vi "filename-manage.vi"(6 "filename pattern":T2, 7 "filename-action":T1=enum."parse", 9 "folder IN":path=path "C:/data/Ultrasound/birdcage/Hg1201/Test", 10 "string IN":string="^(\\s+)(\\d+)_(.*)_(\\d\\d\\d\\d\\d\\d)\\.dat$", 11 "file name IN":string="f027_lsco2_122317.dat") -> (0 "number OUT":dbl=10.0 format="%#_10f", 1 "string OUT":string="^(\\s+)(\\d+)_(.*)_(\\d\\d\\d\\d\\d\\d)\\.dat$", 3 "filename OUT":string)   [LabVIEW 2021]
uses:
  filename-pattern.ctl
  filename-action.ctl
  <vilib>/Utility/libraryn.llb/Check if File or Folder Exists.vi
  <vilib>/regexp/Match Regular Expression.xnode
panel:
  out "offset past match":i32=-1
  out "whole match":string
  out "unique index out":i32
  out "pattern":string="^(\\s+)(\\d+)_(.*)_(\\d\\d\\d\\d\\d\\d)\\.dat$"
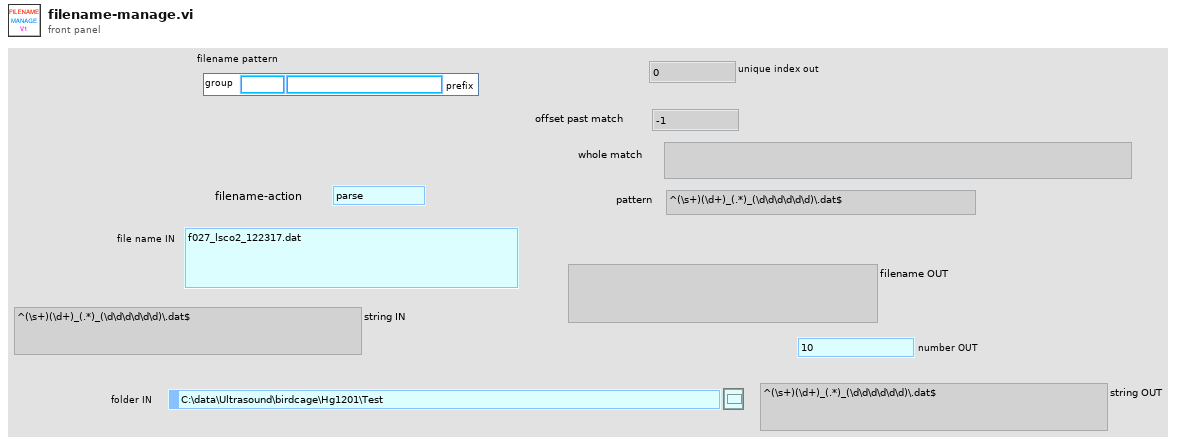
[diagram p1: front panel]
types:
  T1 = typedef "filename-action.ctl" = enum16{"rewrite", "parse", "force pattern", "uniquenum", "get T", "get B", "get ind", "get deg", "get name", "get folder", "get extension", "get basename", "get side", "get setof", "getID", "getIDStock", "remove prefix", "get36thing", "getplain", "getvproj", "getIDStanf", "remove p_c?_"}
  T2 = typedef "filename-pattern.ctl" = cluster{"prefix":string, "group":string}
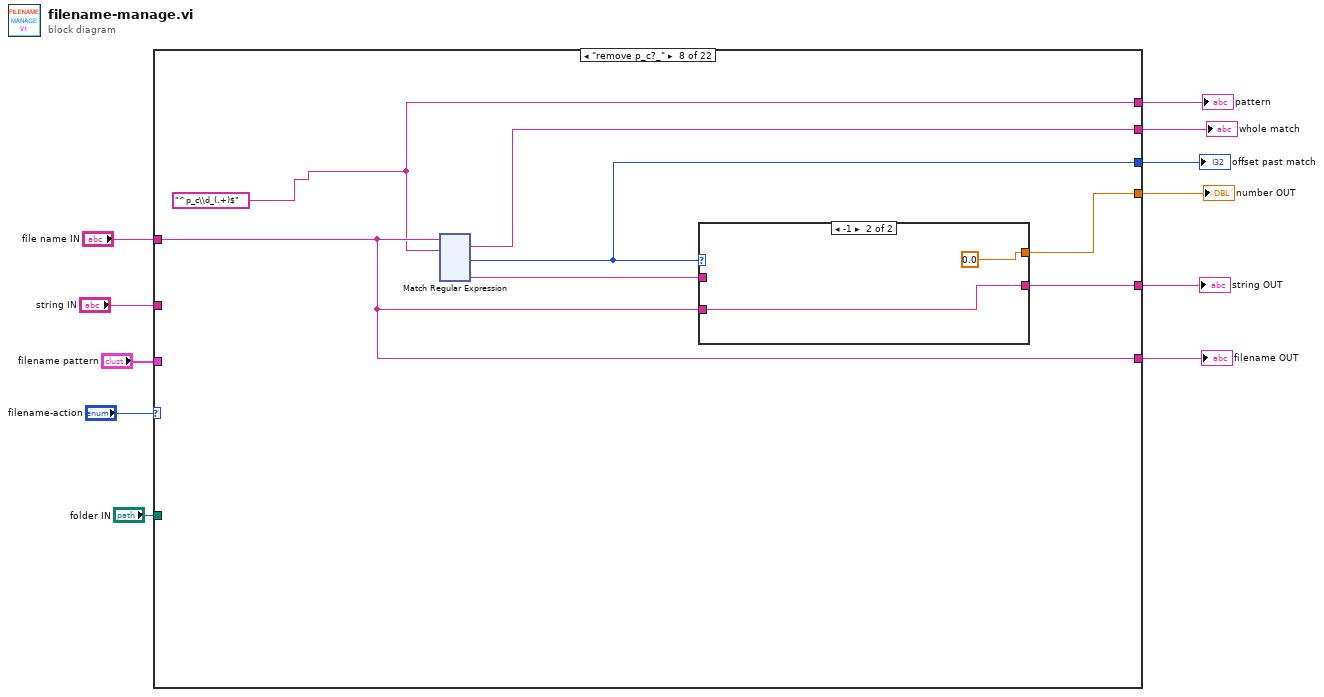
[diagram p0: block diagram]
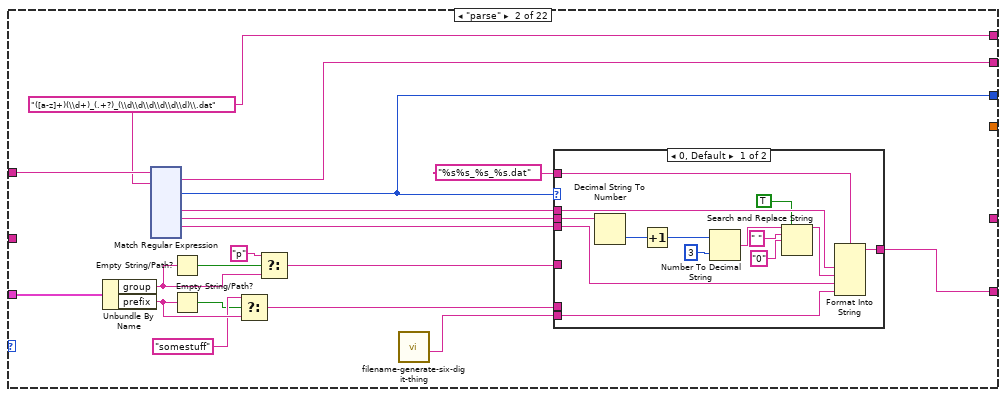
[diagram p3: hidden frame]
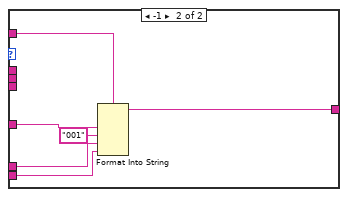
[diagram p4: hidden frame]
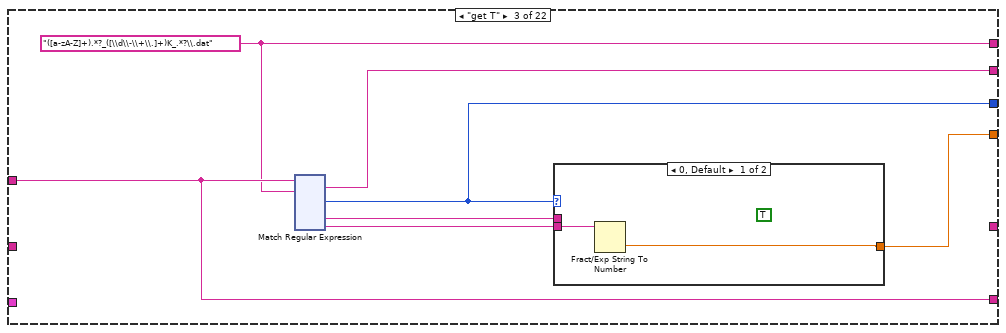
[diagram p5: hidden frame]
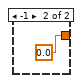
[diagram p6: hidden frame]
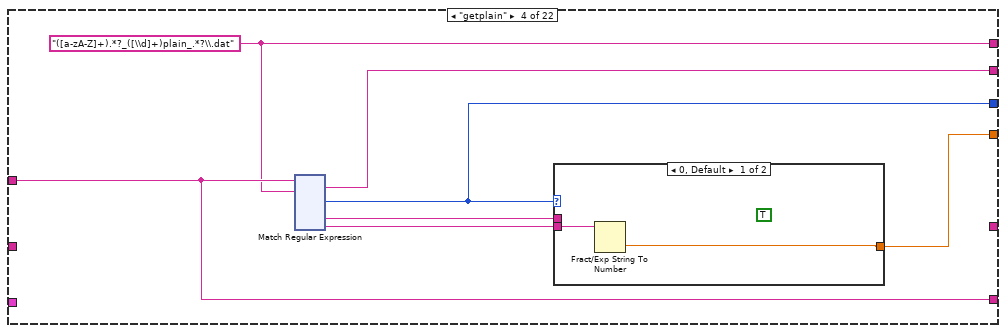
[diagram p7: hidden frame]
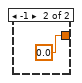
[diagram p8: hidden frame]
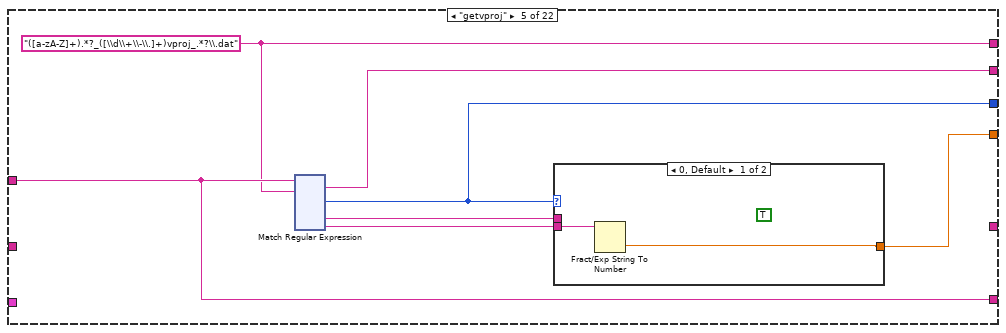
[diagram p9: hidden frame]
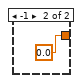
[diagram p10: hidden frame]
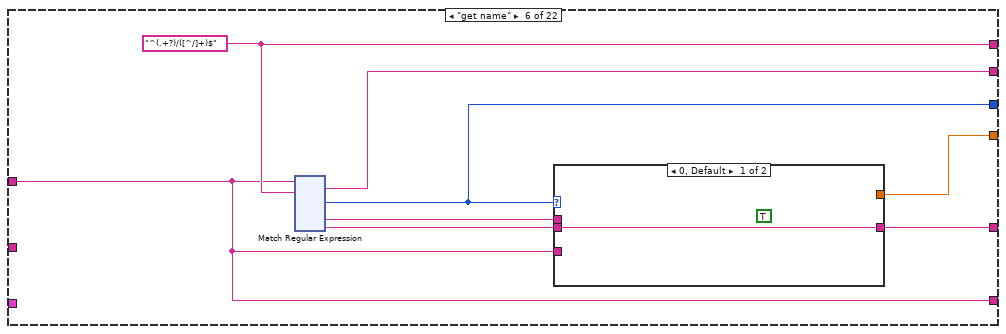
[diagram p11: hidden frame]
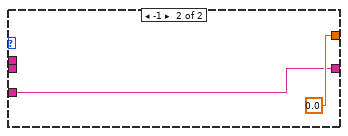
[diagram p12: hidden frame]
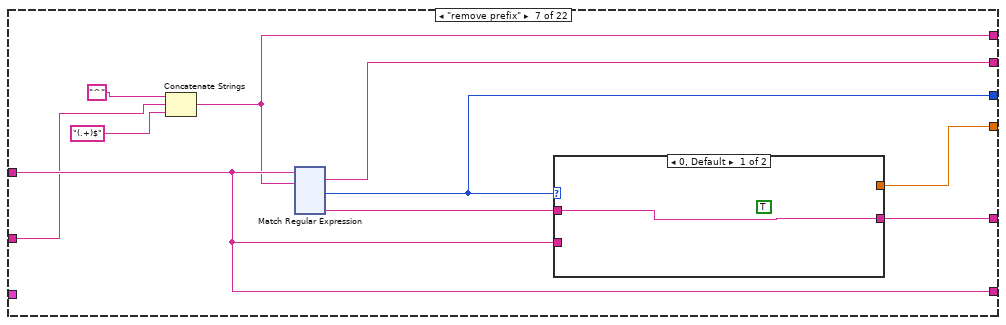
[diagram p13: hidden frame]
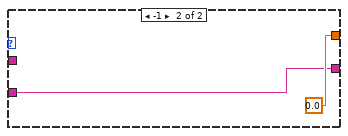
[diagram p14: hidden frame]
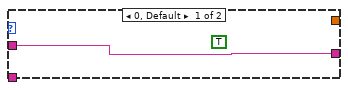
[diagram p15: hidden frame]
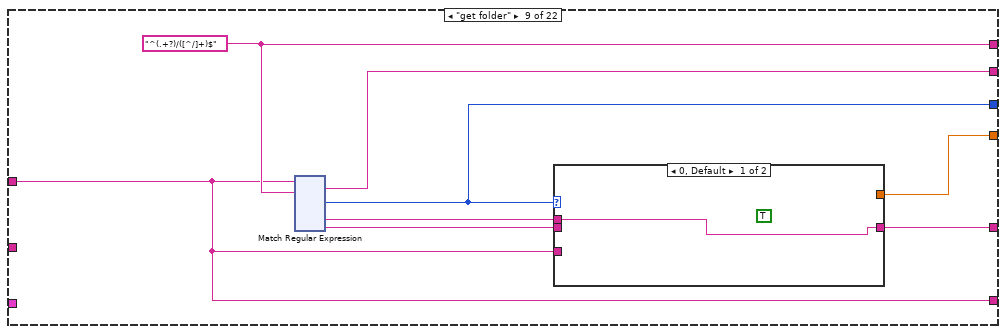
[diagram p16: hidden frame]
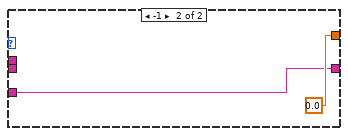
[diagram p17: hidden frame]
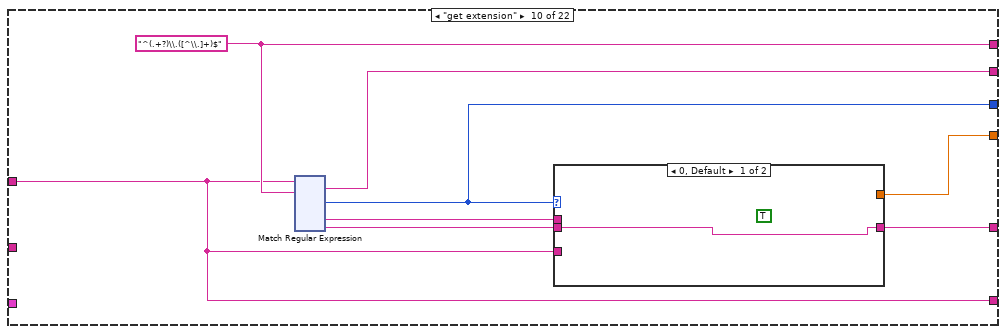
[diagram p18: hidden frame]
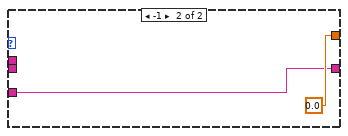
[diagram p19: hidden frame]
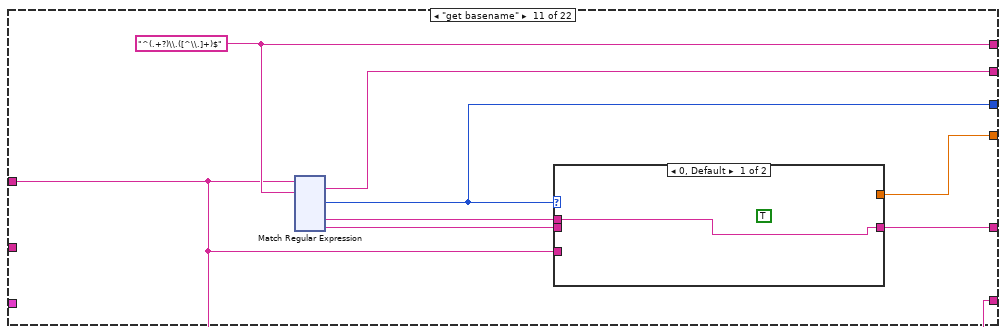
[diagram p20: hidden frame]
diagram:
  n1 = case shown="\"remove p_c?_\"" "filename-action" {
    tunnel: "file name IN" -> [w12 w31 w178 w308 w438 w564 w699 w828 w956 w1087 w1218 w1353 w1483 w1613 w1736 w1863 w1990 w2121 w2253 w2383 w2527 w2691]
    tunnel: "filename pattern" -> [_ w30 _ _ _ _ _ _ _ _ _ _ _ _ _ _ _ _ _ _ w2526 w2690]
    tunnel: [w12 w20 w178 w308 w438 w564 w699 w828 w956 w1087 w1218 w1353 w1483 w1613 w1736 w1863 w1990 w2121 w2253 w2383 w2516 w2681] -> w8
    tunnel: "folder IN" -> [_ _ _ _ _ _ _ _ _ _ _ _ _ _ _ _ _ _ _ _ _ w2676]
    tunnel: [_ _ w177 w307 w437 w569 w703 w832 w961 w1092 w1223 w1352 w1482 _ _ _ _ w2120 w2252 w2382 _ _] -> w6
    tunnel: [_ w13 w176 w306 w436 w568 w702 w831 w960 w1091 w1222 w1351 w1481 w1612 w1740 w1867 w1994 w2119 w2251 w2381 w2509 w2671] -> w5
    tunnel: [_ w14 w175 w305 w435 w567 w701 w830 w959 w1090 w1221 w1350 w1480 w1611 w1739 w1866 w1993 w2118 w2250 w2380 w2510 w2670] -> w4
    tunnel: [_ w15 w174 w304 w434 w566 w695 w827 w958 w1089 w1220 w1349 w1479 w1610 w1737 w1864 w1991 w2117 w2249 w2379 w2511 w2672] -> w3
    tunnel: [_ _ _ _ _ w565 w700 w829 w957 w1088 w1219 _ _ w1609 w1738 w1865 w1992 _ _ _ _ _] -> w2
    tunnel: "string IN" -> [_ _ _ _ _ _ w698 _ _ _ _ _ _ _ _ _ _ _ _ _ _ _]
    frame "rewrite", Default {
    }
    frame "parse" {
      w15 = "([a-z]+)(\\d+)_(.+?)_(\\d\\d\\d\\d\\d\\d)\\.dat" ("format string")
      n2 = Unbundle By Name(w30) -> ("group"=w27:string, "prefix"=w26:string)
      n3 = xnode "Match Regular Expression"("input string"=w31, "regular expression"=w15) -> ("whole match"=w13:string, "offset past match"=w14:i32, "submatch 1"=w18:string, "submatch 2"=w17:string, "submatch 3"=w16:string)  [unwired: 4 in, 4 out]
      n4 = Empty String/Path?(string/path=w27) -> (empty?=w29:bool)
      n5 = Empty String/Path?(string/path=w26) -> (empty?=w24:bool)
      n6 = Select(t="somestuff", s=w24, f=w26) -> (s? t:f=w21:string)
      n7 = Select(t="p", s=w29, f=w27) -> (s? t:f=w22:string)
      n8 = call "filename-generate-six-digit-thing.vi"() -> ("sixdigit"=w19:string)  [unwired: 9 in, 2 out]
      n9 = case shown="0, Default" w14 {
        tunnel: "%s%s_%s_%s.dat" ("format string") -> [w34 w51]
        tunnel: w22 -> [_ w50]
        tunnel: w21 -> [_ w49]
        tunnel: [w44 w48] -> w20
        tunnel: w19 -> [w45 w47]
        tunnel: w18 -> [w43 _]
        tunnel: w17 -> [w42 _]
        tunnel: w16 -> [w33 _]
        frame 0, Default {
          n10 = Decimal String To Number(string=w42) -> (number=w41:i32)  [unwired: 2 in, 1 out]
          n11 = Increment(x=w41) -> (x+1=w40:i32)
          n12 = Number To Decimal String(number=w40, width (-)=i16 3) -> (decimal integer string=w36:string)
          n13 = Search and Replace String(replace all?=TRUE ("replace all? (F)"), input string=w36, search string=" ", replace string="0" ("replace string (\"\")")) -> (result string=w35:string)  [unwired: 4 in, 3 out]
          n14 = Format Into String(format string=w34, w43, w35, w33, w45) -> (resulting string=w44:string)  [unwired: 2 in, 1 out]
        }
        frame -1 {
          n15 = Format Into String(format string=w51, w50, "001" ("input 2"), w49, w47) -> (resulting string=w48:string)  [unwired: 2 in, 1 out]
        }
      }
    }
    frame "get T" {
      w174 = "([a-zA-Z]+).*?_([\\d\\-\\+\\.]+)K_.*?\\.dat" ("format string")
      n16 = xnode "Match Regular Expression"("input string"=w178, "regular expression"=w174) -> ("whole match"=w176:string, "offset past match"=w175:i32, "submatch 1"=w180:string, "submatch 2"=w179:string)  [unwired: 4 in, 3 out]
      n17 = case shown="0, Default" w175 {
        tunnel: [w181 0.0] -> w177
        tunnel: w180 -> [_ _]
        tunnel: w179 -> [w182 _]
        frame 0, Default {
          (unwired) TRUE ("replace all? (F)")
          n18 = Fract/Exp String To Number(string=w182) -> (number=w181:dbl)  [unwired: 3 in, 1 out]
        }
        frame -1 {
        }
      }
    }
    frame "getplain" {
      w304 = "([a-zA-Z]+).*?_([\\d]+)plain_.*?\\.dat" ("format string")
      n19 = xnode "Match Regular Expression"("input string"=w308, "regular expression"=w304) -> ("whole match"=w306:string, "offset past match"=w305:i32, "submatch 1"=w310:string, "submatch 2"=w309:string)  [unwired: 4 in, 3 out]
      n20 = case shown="0, Default" w305 {
        tunnel: [w311 0.0] -> w307
        tunnel: w310 -> [_ _]
        tunnel: w309 -> [w312 _]
        frame 0, Default {
          (unwired) TRUE ("replace all? (F)")
          n21 = Fract/Exp String To Number(string=w312) -> (number=w311:dbl)  [unwired: 3 in, 1 out]
        }
        frame -1 {
        }
      }
    }
    frame "getvproj" {
      w434 = "([a-zA-Z]+).*?_([\\d\\+\\-\\.]+)vproj_.*?\\.dat" ("format string")
      n22 = xnode "Match Regular Expression"("input string"=w438, "regular expression"=w434) -> ("whole match"=w436:string, "offset past match"=w435:i32, "submatch 1"=w440:string, "submatch 2"=w439:string)  [unwired: 4 in, 3 out]
      n23 = case shown="0, Default" w435 {
        tunnel: [w441 0.0] -> w437
        tunnel: w440 -> [_ _]
        tunnel: w439 -> [w442 _]
        frame 0, Default {
          (unwired) TRUE ("replace all? (F)")
          n24 = Fract/Exp String To Number(string=w442) -> (number=w441:dbl)  [unwired: 3 in, 1 out]
        }
        frame -1 {
        }
      }
    }
    frame "get name" {
      w566 = "^(.+?)/([^/]+)$" ("format string")
      n25 = xnode "Match Regular Expression"("input string"=w564, "regular expression"=w566) -> ("whole match"=w568:string, "offset past match"=w567:i32, "submatch 1"=w571:string, "submatch 2"=w570:string)  [unwired: 4 in, 3 out]
      n26 = case shown="0, Default" w567 {
        tunnel: [_ 0.0] -> w569
        tunnel: w571 -> [_ _]
        tunnel: w570 -> [w572 _]
        tunnel: [w572 w573] -> w565
        tunnel: w564 -> [_ w573]
        frame 0, Default {
          (unwired) TRUE ("replace all? (F)")
        }
        frame -1 {
        }
      }
    }
    frame "remove prefix" {
      n27 = Concatenate Strings("^", w698, "(.+)$" ("format string")) -> (w695:string)
      n28 = xnode "Match Regular Expression"("input string"=w699, "regular expression"=w695) -> ("whole match"=w702:string, "offset past match"=w701:i32, "submatch 1"=w704:string)  [unwired: 4 in, 3 out]
      n29 = case shown="0, Default" w701 {
        tunnel: [_ 0.0] -> w703
        tunnel: w704 -> [w705 _]
        tunnel: [w705 w706] -> w700
        tunnel: w699 -> [_ w706]
        frame 0, Default {
          (unwired) TRUE ("replace all? (F)")
        }
        frame -1 {
        }
      }
    }
    frame "remove p_c?_" {
      w827 = "^p_c\\d_(.+)$" ("format string")
      n30 = xnode "Match Regular Expression"("input string"=w828, "regular expression"=w827) -> ("whole match"=w831:string, "offset past match"=w830:i32, "submatch 1"=w833:string)  [unwired: 4 in, 3 out]
      n31 = case shown="-1" w830 {
        tunnel: [_ 0.0] -> w832
        tunnel: w833 -> [w834 _]
        tunnel: [w834 w835] -> w829
        tunnel: w828 -> [_ w835]
        frame 0, Default {
          (unwired) TRUE ("replace all? (F)")
        }
        frame -1 {
        }
      }
    }
    frame "get folder" {
      w958 = "^(.+?)/([^/]+)$" ("format string")
      n32 = xnode "Match Regular Expression"("input string"=w956, "regular expression"=w958) -> ("whole match"=w960:string, "offset past match"=w959:i32, "submatch 1"=w963:string, "submatch 2"=w962:string)  [unwired: 4 in, 3 out]
      n33 = case shown="0, Default" w959 {
        tunnel: [_ 0.0] -> w961
        tunnel: w963 -> [w964 _]
        tunnel: w962 -> [_ _]
        tunnel: [w964 w965] -> w957
        tunnel: w956 -> [_ w965]
        frame 0, Default {
          (unwired) TRUE ("replace all? (F)")
        }
        frame -1 {
        }
      }
    }
    frame "get extension" {
      w1089 = "^(.+?)\\.([^\\.]+)$" ("format string")
      n34 = xnode "Match Regular Expression"("input string"=w1087, "regular expression"=w1089) -> ("whole match"=w1091:string, "offset past match"=w1090:i32, "submatch 1"=w1094:string, "submatch 2"=w1093:string)  [unwired: 4 in, 3 out]
      n35 = case shown="0, Default" w1090 {
        tunnel: [_ 0.0] -> w1092
        tunnel: w1094 -> [_ _]
        tunnel: w1093 -> [w1095 _]
        tunnel: [w1095 w1096] -> w1088
        tunnel: w1087 -> [_ w1096]
        frame 0, Default {
          (unwired) TRUE ("replace all? (F)")
        }
        frame -1 {
        }
      }
    }
    frame "get basename" {
      w1220 = "^(.+?)\\.([^\\.]+)$" ("format string")
      n36 = xnode "Match Regular Expression"("input string"=w1218, "regular expression"=w1220) -> ("whole match"=w1222:string, "offset past match"=w1221:i32, "submatch 1"=w1225:string, "submatch 2"=w1224:string)  [unwired: 4 in, 3 out]
      n37 = case shown="0, Default" w1221 {
        tunnel: [_ 0.0] -> w1223
        tunnel: w1225 -> [w1226 _]
        tunnel: w1224 -> [_ _]
        tunnel: [w1226 w1227] -> w1219
        tunnel: w1218 -> [_ w1227]
        frame 0, Default {
          (unwired) TRUE ("replace all? (F)")
        }
        frame -1 {
        }
      }
    }
    frame "get B" {
      w1349 = "([a-zA-Z]+).*?_([\\d\\-\\+\\.]+)T_.*?\\.dat" ("format string")
      n38 = xnode "Match Regular Expression"("input string"=w1353, "regular expression"=w1349) -> ("whole match"=w1351:string, "offset past match"=w1350:i32, "submatch 1"=w1355:string, "submatch 2"=w1354:string)  [unwired: 4 in, 3 out]
      n39 = case shown="-1" w1350 {
        tunnel: [w1356 0.0] -> w1352
        tunnel: w1355 -> [_ _]
        tunnel: w1354 -> [w1357 _]
        frame 0, Default {
          (unwired) TRUE ("replace all? (F)")
          n40 = Fract/Exp String To Number(string=w1357) -> (number=w1356:dbl)  [unwired: 3 in, 1 out]
        }
        frame -1 {
        }
      }
    }
    frame "get ind" {
      w1479 = "([a-zA-Z]+?).*?_(\\d+)_.*?\\.dat" ("format string")
      n41 = xnode "Match Regular Expression"("input string"=w1483, "regular expression"=w1479) -> ("whole match"=w1481:string, "offset past match"=w1480:i32, "submatch 1"=w1485:string, "submatch 2"=w1484:string)  [unwired: 4 in, 3 out]
      n42 = case shown="0, Default" w1480 {
        tunnel: [w1486 0.0] -> w1482
        tunnel: w1485 -> [_ _]
        tunnel: w1484 -> [w1487 _]
        frame 0, Default {
          (unwired) TRUE ("replace all? (F)")
          n43 = Decimal String To Number(string=w1487) -> (number=w1486:i32)  [unwired: 2 in, 1 out]
        }
        frame -1 {
        }
      }
    }
    frame "getID" {
      w1610 = "([a-zA-Z]+?.*?_\\d+)_.*?\\.dat" ("format string")
      (unwired) "([a-zA-Z]\\d+)_.*?\\.dat" ("format string")
      (unwired) "([a-zA-Z]+?).*?_(\\d+)_.*?\\.dat" ("format string")
      n44 = xnode "Match Regular Expression"("input string"=w1613, "regular expression"=w1610) -> ("whole match"=w1612:string, "offset past match"=w1611:i32, "submatch 1"=w1614:string)  [unwired: 4 in, 3 out]
      n45 = case shown="-1" w1611 {
        tunnel: w1614 -> [w1615 _]
        tunnel: [w1615 "" ("submatch 1")] -> w1609
        frame 0, Default {
          (unwired) TRUE ("replace all? (F)")
        }
        frame -1 {
        }
      }
    }
    frame "getIDStock" {
      w1737 = "(IDS\\d+_\\d+_RAW_cal_).*?\\.dat" ("format string")
      (unwired) "([a-zA-Z]+?.*?_\\d+)_.*?\\.dat" ("format string")
      (unwired) "([a-zA-Z]\\d+)_.*?\\.dat" ("format string")
      (unwired) "([a-zA-Z]+?).*?_(\\d+)_.*?\\.dat" ("format string")
      # "IDS0326_210901_RAW_cal_CeCoIn5_4th_055_Rotation.dat"
      n46 = xnode "Match Regular Expression"("input string"=w1736, "regular expression"=w1737) -> ("whole match"=w1740:string, "offset past match"=w1739:i32, "submatch 1"=w1741:string)  [unwired: 4 in, 3 out]
      n47 = case shown="-1" w1739 {
        tunnel: w1741 -> [w1742 _]
        tunnel: [w1742 "" ("submatch 1")] -> w1738
        frame 0, Default {
          (unwired) TRUE ("replace all? (F)")
        }
        frame -1 {
        }
      }
    }
    frame "getIDStanf" {
      w1864 = "(YTL\\d+_YbVO4_).*?\\.dat" ("format string")
      (unwired) "([a-zA-Z]+?.*?_\\d+)_.*?\\.dat" ("format string")
      (unwired) "([a-zA-Z]\\d+)_.*?\\.dat" ("format string")
      (unwired) "([a-zA-Z]+?).*?_(\\d+)_.*?\\.dat" ("format string")
      # "YTL0229_YbVO4_acchi_12.421K_0.090T_raw_.dat"
      n48 = xnode "Match Regular Expression"("input string"=w1863, "regular expression"=w1864) -> ("whole match"=w1867:string, "offset past match"=w1866:i32, "submatch 1"=w1868:string)  [unwired: 4 in, 3 out]
      n49 = case shown="-1" w1866 {
        tunnel: w1868 -> [w1869 _]
        tunnel: [w1869 "" ("submatch 1")] -> w1865
        frame 0, Default {
          (unwired) TRUE ("replace all? (F)")
        }
        frame -1 {
        }
      }
    }
    frame "get36thing" {
      w1991 = ".*?(\\d\\d\\d_\\d\\d\\d\\d\\d\\d).*?\\.(dat|tdms)" ("format string")
      (unwired) "([a-zA-Z]+?.*?_\\d+)_.*?\\.dat" ("format string")
      (unwired) "([a-zA-Z]\\d+)_.*?\\.dat" ("format string")
      (unwired) "([a-zA-Z]+?).*?_(\\d+)_.*?\\.dat" ("format string")
      # "IDS0326_210901_RAW_cal_CeCoIn5_4th_055_Rotation.dat"
      n50 = xnode "Match Regular Expression"("input string"=w1990, "regular expression"=w1991) -> ("whole match"=w1994:string, "offset past match"=w1993:i32, "submatch 1"=w1995:string)  [unwired: 4 in, 3 out]
      n51 = case shown="-1" w1993 {
        tunnel: w1995 -> [w1996 _]
        tunnel: [w1996 "" ("submatch 1")] -> w1992
        frame 0, Default {
          (unwired) TRUE ("replace all? (F)")
        }
        frame -1 {
        }
      }
    }
    frame "get side" {
      w2117 = "^([a-zA-Z]+?).*?_(ref|sam)_.*?\\.dat$" ("format string")
      n52 = xnode "Match Regular Expression"("input string"=w2121, "regular expression"=w2117) -> ("whole match"=w2119:string, "offset past match"=w2118:i32, "submatch 1"=w2123:string, "submatch 2"=w2122:string)  [unwired: 4 in, 3 out]
      n53 = case shown="0, Default" w2118 {
        tunnel: [w2124 8000] -> w2120
        tunnel: w2123 -> [_ _]
        tunnel: w2122 -> [w2125 _]
        frame 0, Default {
          n54 = case shown="\"sam\", Default" w2125 {
            tunnel: [8000 4000] -> w2124
            frame "sam", Default {
            }
            frame "ref" {
            }
          }
        }
        frame -1 {
        }
      }
    }
    frame "get setof" {
      w2249 = "[a-zA-Z]+?.*?_(Tdep|Tset|Bdep|Bset)_.*?\\.dat" ("format string")
      # "Tset = 1\nBset = 2"
      n55 = xnode "Match Regular Expression"("input string"=w2253, "regular expression"=w2249) -> ("whole match"=w2251:string, "offset past match"=w2250:i32, "submatch 1"=w2254:string)  [unwired: 4 in, 3 out]
      n56 = case shown="0, Default" w2250 {
        tunnel: [w2256 1.0] -> w2252
        tunnel: w2254 -> [w2255 _]
        frame 0, Default {
          (unwired) TRUE ("replace all? (F)")
          n57 = case shown="\"Tdep\", \"Tset\", Default" w2255 {
            tunnel: [1 2] -> w2256
            frame "Tdep", "Tset", Default {
            }
            frame "Bdep", "Bset" {
            }
          }
        }
        frame -1 {
        }
      }
    }
    frame "get deg" {
      w2379 = "([a-zA-Z]+)_([\\d\\-\\+\\.]+)deg.*?" ("format string")
      (unwired) "([a-zA-Z]+?).*?_(\\d\\d\\d)_.*?\\.dat" ("format string")
      n58 = xnode "Match Regular Expression"("input string"=w2383, "regular expression"=w2379) -> ("whole match"=w2381:string, "offset past match"=w2380:i32, "submatch 1"=w2385:string, "submatch 2"=w2384:string)  [unwired: 4 in, 3 out]
      n59 = case shown="0, Default" w2380 {
        tunnel: [w2386 0.0] -> w2382
        tunnel: w2385 -> [_ _]
        tunnel: w2384 -> [w2387 _]
        frame 0, Default {
          (unwired) TRUE ("replace all? (F)")
          n60 = Decimal String To Number(string=w2387) -> (number=w2386:i32)  [unwired: 2 in, 1 out]
        }
        frame -1 {
        }
      }
    }
    frame "force pattern" {
      w2511 = "([a-z]+)(\\d+)_(.+?)_(\\d\\d\\d\\d\\d\\d)\\.dat" ("format string")
      n61 = Unbundle By Name(w2526) -> ("group"=w2523:string, "prefix"=w2522:string)
      n62 = xnode "Match Regular Expression"("input string"=w2527, "regular expression"=w2511) -> ("whole match"=w2509:string, "offset past match"=w2510:i32, "submatch 1"=w2514:string, "submatch 2"=w2513:string, "submatch 3"=w2512:string)  [unwired: 4 in, 4 out]
      n63 = Empty String/Path?(string/path=w2523) -> (empty?=w2525:bool)
      n64 = Empty String/Path?(string/path=w2522) -> (empty?=w2520:bool)
      n65 = Select(t="somestuff", s=w2520, f=w2522) -> (s? t:f=w2517:string)
      n66 = call "filename-generate-six-digit-thing.vi"() -> ("sixdigit"=w2515:string)  [unwired: 9 in, 2 out]
      n67 = Select(t="p", s=w2525, f=w2523) -> (s? t:f=w2518:string)
      n68 = case shown="0, Default" w2510 {
        tunnel: "%s%s_%s_%s.dat" ("format string") -> [w2531 w2547]
        tunnel: w2518 -> [w2530 w2546]
        tunnel: w2517 -> [w2529 w2545]
        tunnel: [w2540 w2544] -> w2516
        tunnel: w2515 -> [w2541 w2543]
        tunnel: w2514 -> [_ _]
        tunnel: w2513 -> [w2539 _]
        tunnel: w2512 -> [_ _]
        frame 0, Default {
          n69 = Decimal String To Number(string=w2539) -> (number=w2538:i32)  [unwired: 2 in, 1 out]
          n70 = Increment(x=w2538) -> (x+1=w2537:i32)
          n71 = Number To Decimal String(number=w2537, width (-)=i16 3) -> (decimal integer string=w2533:string)
          n72 = Search and Replace String(replace all?=TRUE ("replace all? (F)"), input string=w2533, search string=" ", replace string="0" ("replace string (\"\")")) -> (result string=w2532:string)  [unwired: 4 in, 3 out]
          n73 = Format Into String(format string=w2531, w2530, w2532, w2529, w2541) -> (resulting string=w2540:string)  [unwired: 2 in, 1 out]
        }
        frame -1 {
          n74 = Format Into String(format string=w2547, w2546, "001" ("input 2"), w2545, w2543) -> (resulting string=w2544:string)  [unwired: 2 in, 1 out]
        }
      }
    }
    frame "uniquenum" {
      w2672 = "([a-z]+)(\\d+)_(.+?)_(\\d\\d\\d\\d\\d\\d)\\.dat" ("format string")
      n75 = Unbundle By Name(w2690) -> ("group"=w2687:string, "prefix"=w2686:string)
      n76 = call "file -- 9w path.vi"("sweep folder"=w2676) -> ("9w path"=w2675:path)  [unwired: 10 in]
      n77 = xnode "Match Regular Expression"("input string"=w2691, "regular expression"=w2672) -> ("whole match"=w2671:string, "offset past match"=w2670:i32, "submatch 1"=w2679:string, "submatch 2"=w2678:string, "submatch 3"=w2677:string)  [unwired: 4 in, 4 out]
      n78 = Empty String/Path?(string/path=w2687) -> (empty?=w2689:bool)
      n79 = Empty String/Path?(string/path=w2686) -> (empty?=w2684:bool)
      n80 = Select(t="somestuff", s=w2684, f=w2686) -> (s? t:f=w2682:string)
      n81 = call "filename-generate-six-digit-thing.vi"() -> ("sixdigit"=w2680:string)  [unwired: 9 in, 2 out]
      n82 = Select(t="p", s=w2689, f=w2687) -> (s? t:f=w2674:string)
      n83 = call "file -- get unique increment name.vi"("prefix"=w2674, "9w folder path"=w2675) -> ("unique index out"=w2673:i32)  [unwired: 9 in]
      "unique index out" <- w2673
      n84 = case shown="0, Default" w2670 {
        tunnel: "%s%s_%s_%s.dat" ("format string") -> [w2696 w2709]
        tunnel: w2674 -> [w2695 w2708]
        tunnel: w2682 -> [w2694 w2707]
        tunnel: [w2702 w2706] -> w2681
        tunnel: w2680 -> [w2703 w2705]
        tunnel: w2679 -> [_ _]
        tunnel: w2678 -> [_ _]
        tunnel: w2677 -> [_ _]
        tunnel: w2673 -> [w2693 _]
        frame 0, Default {
          n85 = Number To Decimal String(number=w2693, width (-)=i16 3) -> (decimal integer string=w2698:string)
          n86 = Search and Replace String(replace all?=TRUE ("replace all? (F)"), input string=w2698, search string=" ", replace string="0" ("replace string (\"\")")) -> (result string=w2697:string)  [unwired: 4 in, 3 out]
          n87 = Format Into String(format string=w2696, w2695, w2697, w2694, w2703) -> (resulting string=w2702:string)  [unwired: 2 in, 1 out]
        }
        frame -1 {
          n88 = Format Into String(format string=w2709, w2708, "001" ("input 2"), w2707, w2705) -> (resulting string=w2706:string)  [unwired: 2 in, 1 out]
        }
      }
    }
  }
  "filename OUT" <- w8
  "number OUT" <- w6
  "whole match" <- w5
  "offset past match" <- w4
  "pattern" <- w3
  "string OUT" <- w2
